vi "setValue.vi"(8 "error in (no error)":errorcluster, 10 "Value":string, 11 "XML Tree in":refnum<class "XML Tree.lvclass">) -> (0 "error out":errorcluster, 3 "XML Tree out":refnum<class "XML Tree.lvclass">)   [LabVIEW 2013, in "XML Tree.lvclass"]
uses:
  XML Tree.lvclass
  XML Tree.lvclass/XML Tree.ctl
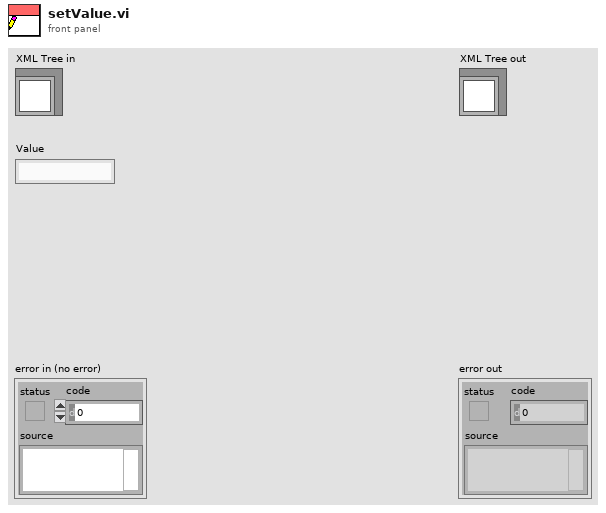
[diagram p1: front panel]
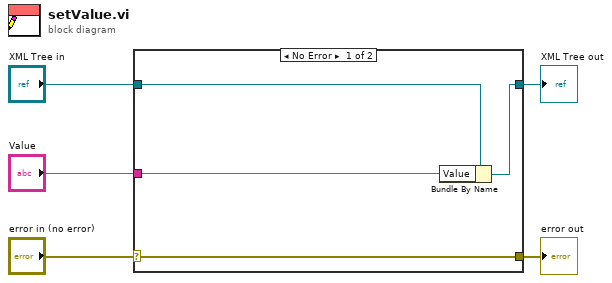
[diagram p0: block diagram]
diagram:
  n1 = case shown="No Error" "error in (no error)" {
    selector: "error in (no error)" -> [w9 w10]
    tunnel: [w9 w10] -> w4
    tunnel: [w7 w11] -> w2
    tunnel: "XML Tree in" -> [w8 w11]
    tunnel: "Value" -> [w6 _]
    frame No Error {
      n2 = Bundle By Name(cluster=w8, "Value"=w6) -> (w7:refnum<class "XML Tree.lvclass">)
    }
    frame Error {
    }
  }
  "error out" <- w4
  "XML Tree out" <- w2
